vi "jl-script abs path.vi"(8 "error in (no error)":errorcluster, 10 "Base path (not a path)":path=path "", 11 "Julia user functions script":path) -> (0 "error out":errorcluster, 3 "script abs path":path)   [LabVIEW 2018, in "LV2Julia_core.lvlib"]
doc: "If abs path is connected, this VI only checks if this file exists and puts the path through.\nFor a relative path, the abs path is constructed using the base path."
uses:
  LV2Julia_core.lvlib
  <vilib>/Utility/error.llb/Error Cluster From Error Code.vi
  <vilib>/ErrorRing/Error Ring.xnode
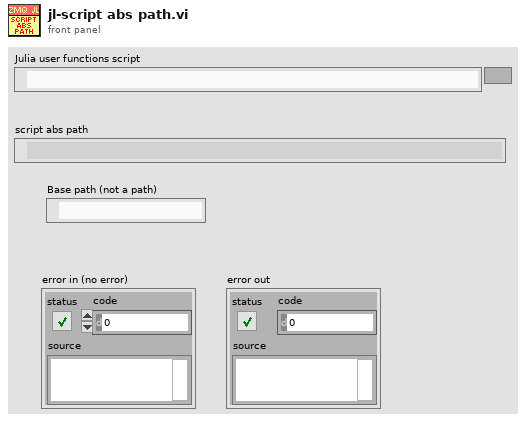
[diagram p1: front panel]
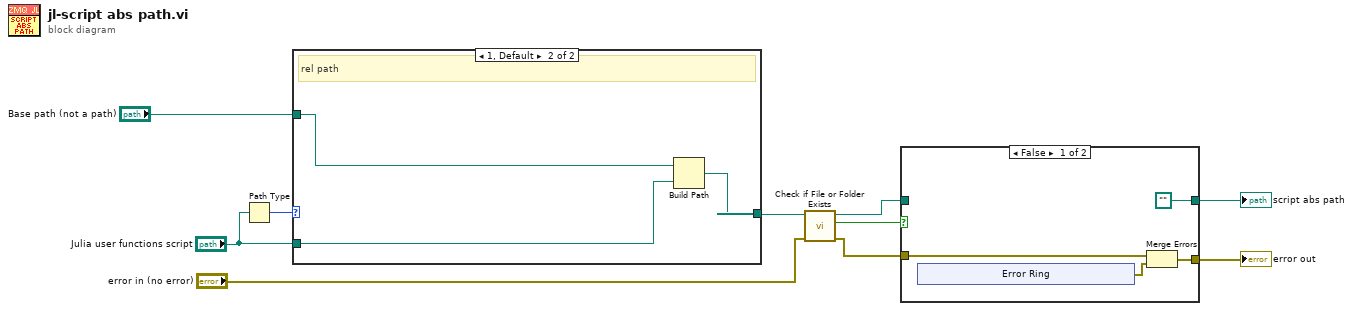
[diagram p0: block diagram]
diagram:
  n1 = Path Type(1:"Julia user functions script") -> (0:w3:i16)
  n2 = case shown="1, Default" w3 {
    tunnel: [w11 w14] -> w8
    tunnel: "Julia user functions script" -> [w11 w13]
    tunnel: "Base path (not a path)" -> [_ w12]
    frame 0 {
      # "abs path"
    }
    frame 1, Default {
      # "rel path"
      n3 = Build Path(base path=w12, name or relative path=w13) -> (appended path=w14:path)
    }
  }
  n4 = call <vilib>:"Check if File or Folder Exists.vi"("error in (no error)"="error in (no error)", "path"=w8) -> ("error out"=w7:errorcluster, "file or folder exists?"=w10:bool, "dup path"=w9:path)  [unwired: 7 in]
  n5 = case shown="False" w10 {
    tunnel: w9 -> [_ w25]
    tunnel: [w17 w24] -> w4
    tunnel: w7 -> [w16 w24]
    tunnel: [path "" w25] -> w5
    frame False {
      n6 = xnode "Error Ring"() -> ("error out"=w18:errorcluster)
      n7 = Merge Errors(w16, w18) -> (w17:errorcluster)
    }
    frame True {
      # "script file exists"
    }
  }
  "script abs path" <- w5
  "error out" <- w4
